vi "Dummy Target VI.vi"() -> ()   [LabVIEW 2020]
panel:
  out "Numeric out":i32
  in  "Numeric in":i32
  out "error out":errorcluster
  in  "error in":errorcluster
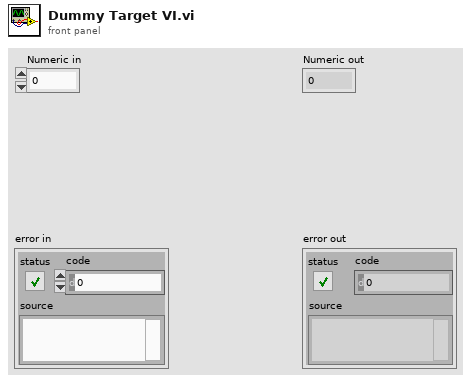
[diagram p1: front panel]
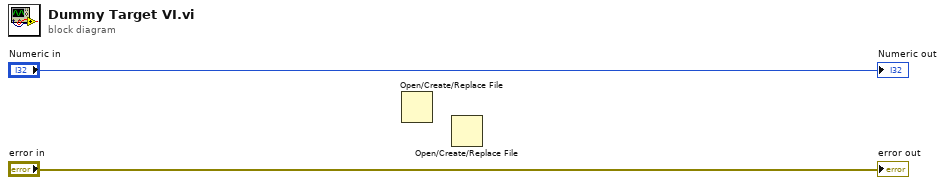
[diagram p0: block diagram]
diagram:
  n1 = Open/Create/Replace File() -> ()  [unwired: 6 in, 3 out]
  n2 = Open/Create/Replace File() -> ()  [unwired: 6 in, 3 out]
  "error out" <- "error in"
  "Numeric out" <- "Numeric in"
